vi "ToRepo.vi"(8 "error in":errorcluster, 9 "to repo cluster":T1, 10 "repository in":refnum<class "CEF_Repository.lvclass">, 11 "CEF_Serialize node in":refnum<class "CEF_serializable node.lvclass">) -> (0 "error out":errorcluster, 2 "repository out":refnum<class "CEF_Repository.lvclass">, 3 "CEF_Serialize node out":refnum<class "CEF_serializable node.lvclass">)   [LabVIEW 2025, in "CEF.lvlib" / "CEF_serializable node.lvclass"]
doc: "Transfers the information from the tree node into the repo. How it is stored in the repo depends on the Repo. For children of NISE_CEF_serializable node.lvclass, the parent method must be called to maintain the chain of serialization. If it is not called, the repo generation will fail.Copyright 2017 National Instruments Corporation\n\nLicensed under the Apache License, Version 2.0 (the \"License\"); you may not use this file except in compliance with the License. You may obtain a copy of the License at http://www.apache.org/licenses/LICENSE-2.0\nUnless required by applicable law or agreed to in writing, software distributed under the License is distributed on an \"AS IS\" BASIS, WITHOUT WARRANTIES OR CONDITIONS OF ANY KIND, either express or implied. See the License for the specific language governing permissions and limitations under the License."
uses:
  CEF_serializable node.lvclass
  Repository/CEF_Repository.lvclass
  Node/ToRepoCluster.ctl
  hierarchy repo/CEF_HierarchyRepo.lvclass
  C:/Working copy/tss/Plugin/CEF/Repository/CEF_Repository.lvclass
  serializable configuration/CEF_serializable configuration.lvclass/CEF_serializable configuration.ctl
  <vilib>/Utility/LVClass/Get LV Class Name.vi
  error generator/CEF_error generator.vi
  Node/CEF_Node.lvclass
  serializable configuration/CEF_serializable configuration.lvclass
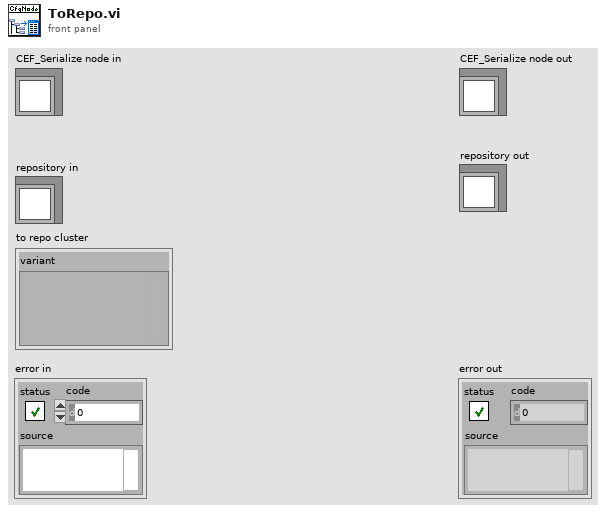
[diagram p1: front panel]
types:
  T1 = typedef "CEF.lvlib/CEF_Node.lvclass/ToRepoCluster.ctl" = cluster{"variant":variant}
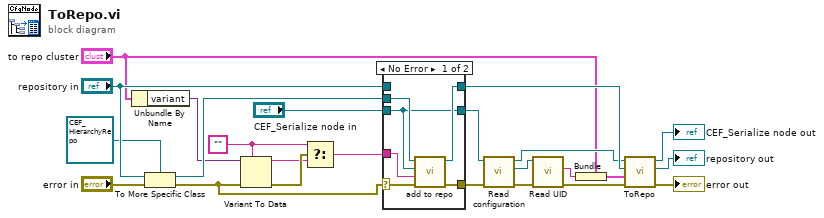
[diagram p0: block diagram]
diagram:
  w2 = ""
  n1 = Unbundle By Name("to repo cluster") -> ("variant"=w15:variant)
  n2 = To More Specific Class(target class=refnum<class "CEF_HierarchyRepo.lvclass"> refnum ("CEF_HierarchyRepo.lvclass"), reference="repository in", error in="error in") -> (specific class reference=w20:refnum<class "CEF_HierarchyRepo.lvclass">, error out=w5:errorcluster)
  n3 = Variant To Data(error in=w5, type=w2, Variant=w15) -> (data=w3:string, error out=w4:errorcluster)
  n4 = Select(t=w2, s=w4, f=w3) -> (s? t:f=w1:string)
  n5 = case shown="No Error" w5 {
    selector: w5 -> [w27 w32]
    tunnel: "repository in" -> [_ w33]
    tunnel: [w29 w33] -> w16
    tunnel: [w28 w32] -> w10
    tunnel: "CEF_Serialize node in" -> [w26 w31]
    tunnel: [w26 w31] -> w11
    tunnel: w20 -> [w30 _]
    tunnel: w1 -> [w25 _]
    frame No Error {
      n6 = call-dynamic "add to repo.vi"("error in"=w27, "parent"=w25, "serializable node"=w26, "CEF_HierarchyRepo in"=w30) -> ("error out"=w28:errorcluster, "CEF_HierarchyRepo out"=w29:refnum<class "CEF_HierarchyRepo.lvclass">)  [unwired: 6 in]
    }
    frame Error {
    }
  }
  n7 = call-dynamic "Read configuration.vi"("error in"=w10, "CEF_serializable node in"=w11) -> ("error out"=w9:errorcluster, "CEF Configuration"=w13:refnum<class "CEF_serializable configuration.lvclass">, "CEF_serializable node out"=w12:refnum<class "CEF_serializable node.lvclass">)  [unwired: 7 in]
  n8 = call "Read UID.vi"("error in"=w9, "CEF_Configuration in"=w13) -> ("error out"=w14:errorcluster, "instance id"=w8:string)  [unwired: 7 in, 1 out]
  n9 = Bundle(cluster="to repo cluster", "variant"=w8) -> (w7:T1)
  n10 = call-parent "ToRepo.vi"("error in"=w14, "to repo cluster"=w7, "repository in"=w16, "CEF_Node in"=w12) -> ("error out"=→"error out":errorcluster, "repository out"=→"repository out":refnum<class "CEF_Repository.lvclass">, "CEF_Node out"=→"CEF_Serialize node out":refnum<class "CEF_serializable node.lvclass">)  [unwired: 5 in]
